vi "Rebin Image.vi"(6 "Dest Binning":i32, 7 "Src Binning":i32, 8 "error in (no error)":errorcluster, 9 "Scale Intensity? (F)":bool, 10 "Dest Image":T1, 11 "Src Image":T1) -> (0 "error out":errorcluster, 3 "Dest Image":T1)   [LabVIEW 2021, in "Image.lvlib"]
doc: "If Dest Binning is <= 0, the Src Image is copied unchanged into the Dest Image"
uses:
  Image.lvlib
  <vilib>/vision/Image Controls.llb/IMAQ Image.ctl
  8a60cfbd-50d1-42da-9e72-1887c40cfc35.vi
  Time/High Resolution Timing.vi
  <vilib>/vision/NI_Vision_Development_Module.lvlib
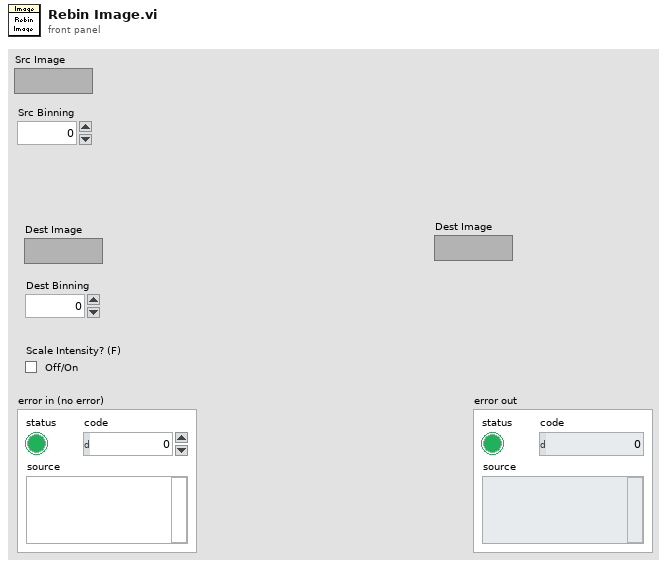
[diagram p1: front panel]
types:
  T1 = typedef "IMAQ Image.ctl" = refnum<image>
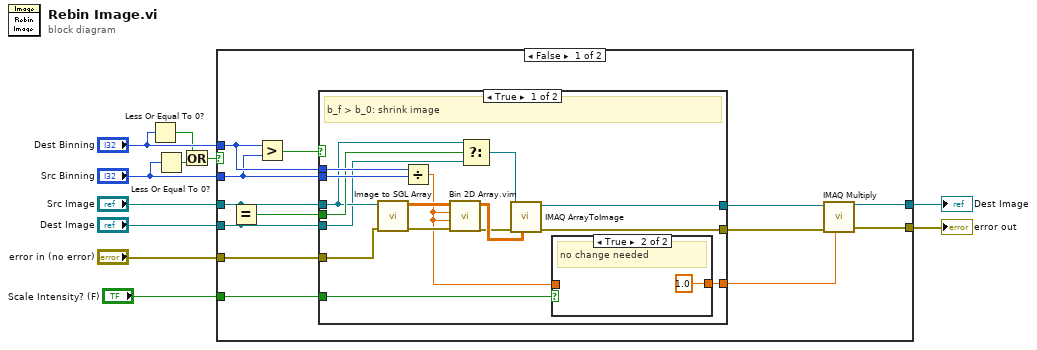
[diagram p0: block diagram]
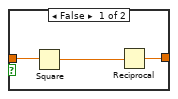
[diagram p2: hidden frame]
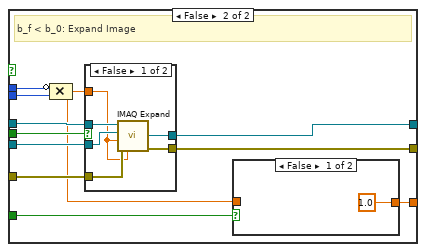
[diagram p3: hidden frame]
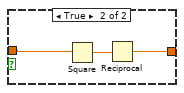
[diagram p4: hidden frame]
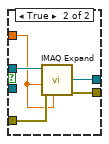
[diagram p5: hidden frame]
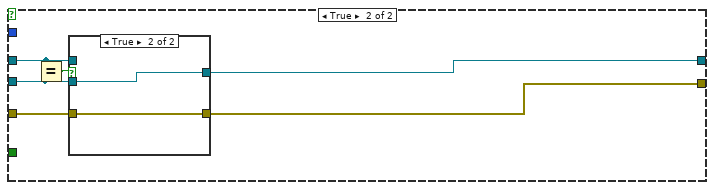
[diagram p6: hidden frame]
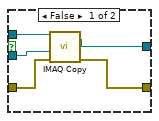
[diagram p7: hidden frame]
diagram:
  n1 = Less Or Equal To 0?(x="Dest Binning") -> (x <= 0?=w3:bool)
  n2 = Less Or Equal To 0?(x="Src Binning") -> (x <= 0?=w4:bool)
  n3 = Or(x=w3, y=w4) -> (x .or. y?=w2:bool)
  n4 = case shown="False" w2 {
    tunnel: [w18 w74] -> w11
    tunnel: "error in (no error)" -> [w14 w75]
    tunnel: [w19 w76] -> w9
    tunnel: "Src Image" -> [w24 w73]
    tunnel: "Dest Image" -> [w23 w72]
    tunnel: "Dest Binning" -> [w17 _]
    tunnel: "Src Binning" -> [w16 _]
    tunnel: "Scale Intensity? (F)" -> [w13 _]
    frame False {
      n5 = Equal?(x=w24, y=w23) -> (x = y?=w22:bool)
      n6 = Greater?(x=w17, y=w16) -> (0:w15:bool)
      n7 = case shown="True" w15 {
        tunnel: w23 -> [w29 w55]
        tunnel: w24 -> [w30 w52]
        tunnel: [w33 w54] -> w21
        tunnel: [w32 w53] -> w20
        tunnel: w17 -> [w37 w51]
        tunnel: w16 -> [w36 w50]
        tunnel: w14 -> [w40 w49]
        tunnel: w22 -> [w31 w48]
        tunnel: w13 -> [w27 w47]
        tunnel: [w26 w45] -> w12
        frame True {
          # "b_f > b_0: shrink image"
          n8 = call "Image to SGL Array.vi"("error in (no error)"=w40, "Image"=w30) -> ("error out"=w38:errorcluster, "Image Pixels (Float)"=w39:sgl[][])  [unwired: 6 in, 2 out]
          n9 = Divide(x=w37, y=w36) -> (x/y=w25:dbl)
          n10 = call "Bin 2D Array.vim"("Error In"=w38, "Y Bin (1)"=w25, "X Bin (1)"=w25, "Array"=w39) -> ("Error Out"=w34:errorcluster, "Binned Array"=w35:sgl[][])  [unwired: 2 in, 4 out]
          n11 = Select(t=w30, s=w31, f=w29) -> (s? t:f=w28:T1)
          n12 = call "IMAQ ArrayToImage"("Image Pixels (Float)"=w35, "error in (no error)"=w34, "Image"=w28) -> ("error out"=w32:errorcluster, "Image Out"=w33:T1)  [unwired: 7 in]
          n13 = case shown="True" w27 {
            tunnel: [w41 1.0 ("Constant")] -> w26
            tunnel: w25 -> [w43 _]
            frame False {
              n14 = Square(x=w43) -> (x^2=w42:dbl)
              n15 = Reciprocal(x=w42) -> (1/x=w41:dbl)
            }
            frame True {
              # "no change needed"
            }
          }
        }
        frame False {
          # "b_f < b_0: Expand Image"
          n16 = Compound Arithmetic op=MULTIPLY(invert w51, w50) -> (w46:dbl)
          n17 = case shown="False" w48 {
            tunnel: w55 -> [w65 _]
            tunnel: [w64 w70] -> w54
            tunnel: [w63 w69] -> w53
            tunnel: w52 -> [w62 w68]
            tunnel: w46 -> [w60 w66]
            tunnel: w49 -> [w61 w67]
            frame False {
              n18 = call "IMAQ Expand"("Y Duplication Step"=w60, "error in (no error)"=w61, "X Duplication Step"=w60, "Image Dst"=w65, "Image Src"=w62) -> ("error out"=w63:errorcluster, "Image Dst Out"=w64:T1)  [unwired: 5 in]
            }
            frame True {
              n19 = call "IMAQ Expand"("Y Duplication Step"=w66, "error in (no error)"=w67, "X Duplication Step"=w66, "Image Src"=w68) -> ("error out"=w69:errorcluster, "Image Dst Out"=w70:T1)  [unwired: 6 in]
            }
          }
          n20 = case shown="False" w47 {
            tunnel: w46 -> [_ w59]
            tunnel: [1.0 w57] -> w45
            frame False {
            }
            frame True {
              n21 = Square(x=w59) -> (x^2=w58:dbl)
              n22 = Reciprocal(x=w58) -> (1/x=w57:dbl)
            }
          }
        }
      }
      n23 = call "IMAQ Multiply"("Image Src A"=w21, "Constant"=w12, "error in (no error)"=w20) -> ("Image Dst Out"=w19:T1, "error out"=w18:errorcluster)  [unwired: 4 in]
    }
    frame True {
      n24 = Equal?(x=w73, y=w72) -> (x = y?=w71:bool)
      n25 = case shown="True" w71 {
        tunnel: [w81 w82] -> w76
        tunnel: w75 -> [w80 w83]
        tunnel: [w79 w83] -> w74
        tunnel: w73 -> [w78 _]
        tunnel: w72 -> [w77 w82]
        frame False {
          n26 = call "IMAQ Copy"("error in (no error)"=w80, "Image Dst"=w77, "Image Src"=w78) -> ("error out"=w79:errorcluster, "Image Dst Out"=w81:T1)  [unwired: 3 in]
        }
        frame True {
        }
      }
    }
  }
  "error out" <- w11
  "Dest Image" <- w9
